vi "Build MVS command substring.vi"(2 "Affected axes":string[](array[string]), 3 "Position values":dbl[](array[numeric]) format="%.8f", 4 "No.of digits\nfor Pos. values":i16=4, 6 "Step size":dbl[](array[numeric]) format="%.6f", 7 "No.of digits\nfor Step size":i16=4, 8 "Delay time":dbl[](array[numeric])) -> (14 "Command substring":string)   [LabVIEW 2026]
doc: "This VI builds a command substring for the MVS command by combining axis identifier and three parameters."
panel:
  # "This vi builds a command substring for the MVS command by combining axis identifier and three parameters."
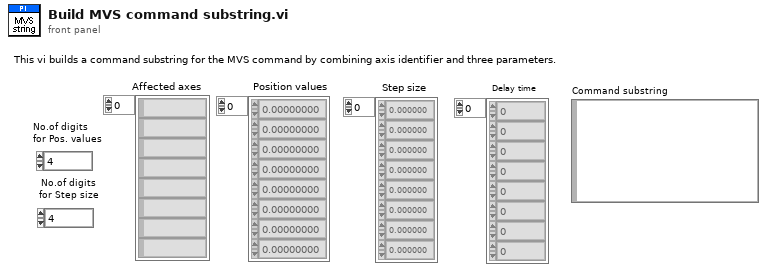
[diagram p1: front panel]
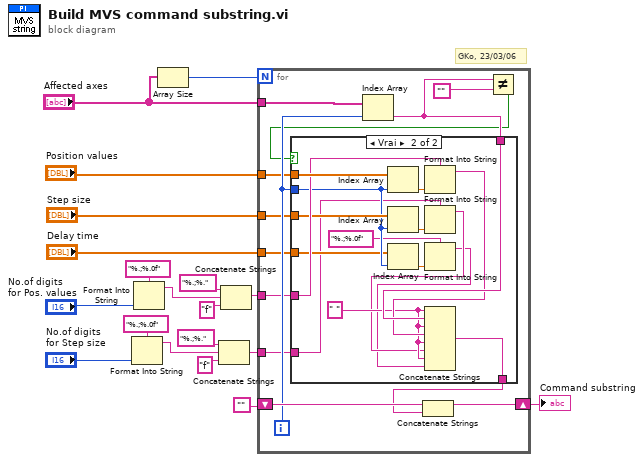
[diagram p0: block diagram]
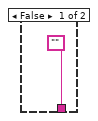
[diagram p2: hidden frame]
diagram:
  # "GKo, 23/03/06"
  n1 = Format Into String(format string="%.;%.0f" ("Format String"), "No.of digits\nfor Step size") -> (resulting string=w5:string)  [unwired: 2 in, 1 out]
  n2 = Format Into String(format string="%.;%.0f" ("Format String"), "No.of digits\nfor Pos. values") -> (resulting string=w10:string)  [unwired: 2 in, 1 out]
  n3 = Array Size(array="Affected axes") -> (size(s)=w9:i32)
  n4 = Concatenate Strings("%.;%." ("Format String"), w5, "f" ("Format String")) -> (w1:string)
  n5 = Concatenate Strings("%.;%." ("Format String"), w10, "f" ("Format String")) -> (w13:string)
  n6 = for {
    N: w9 -> [_]
    shift-right: [w31] -> w18
    shift-left: "" -> [w32]
    tunnel: "Position values" -> [w28]
    tunnel: w13 -> [w27]
    tunnel: "Affected axes" -> [w26]
    tunnel: "Step size" -> [w22]
    tunnel: "Delay time" -> [w21]
    tunnel: w1 -> [w20]
    i -> [w29]
    n7 = Index Array(array=w26, index=w29) -> (element=w25:string)
    n8 = Not Equal?(x=w25, y="") -> (x != y?=w23:bool)
    n9 = case shown="Vrai" w23 {
      tunnel: ["" w49] -> w30
      tunnel: w29 -> [_ w40]
      tunnel: w28 -> [_ w48]
      tunnel: w27 -> [_ w47]
      tunnel: w25 -> [_ w46]
      tunnel: w22 -> [_ w42]
      tunnel: w21 -> [_ w39]
      tunnel: w20 -> [_ w38]
      frame False {
      }
      frame True {
        w36 = " " ("Substring")
        n10 = Index Array(array=w48, index=w40) -> (element=w44:dbl)
        n11 = Index Array(array=w42, index=w40) -> (element=w43:dbl)
        n12 = Index Array(array=w39, index=w40) -> (element=w41:dbl)
        n13 = Format Into String(format string=w47, w44) -> (resulting string=w45:string)  [unwired: 2 in, 1 out]
        n14 = Format Into String(format string=w38, w43) -> (resulting string=w35:string)  [unwired: 2 in, 1 out]
        n15 = Format Into String(format string="%.;%.0f" ("Format String"), w41) -> (resulting string=w34:string)  [unwired: 2 in, 1 out]
        n16 = Concatenate Strings(w36, w46, w36, w45, w36, w35, w36, w34) -> (w49:string)
      }
    }
    n17 = Concatenate Strings(w32, w30) -> (w31:string)
  }
  "Command substring" <- w18
